vi "mWmotor_Set_Driver_current.vi"(8 "error in (no error)":errorcluster, 10 "Boolean":bool, 11 "VISA resource name":refnum<visa-resource-name>) -> (0 "error out":errorcluster, 3 "VISA resource name out":refnum<visa-resource-name>)   [LabVIEW 2019]
panel:
  in  "milliseconds to wait":u32=100
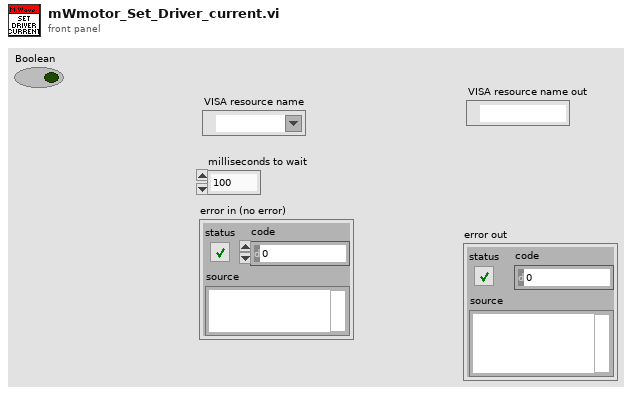
[diagram p1: front panel]
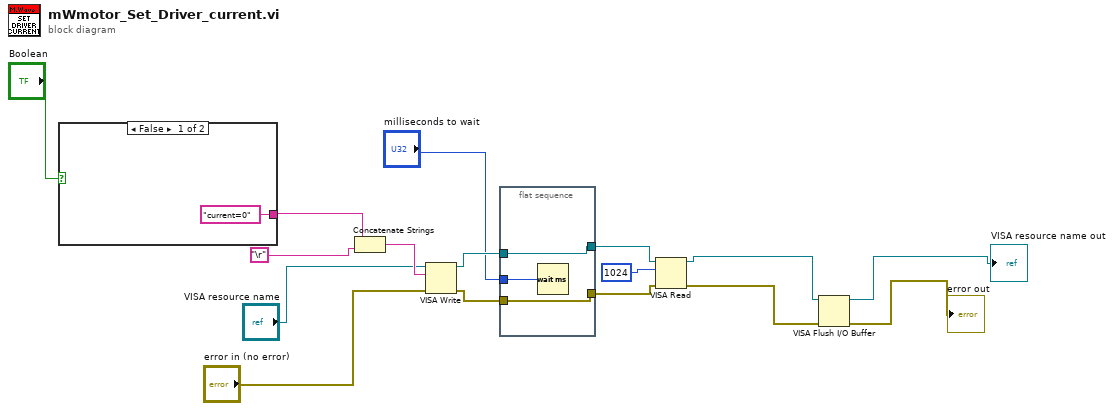
[diagram p0: block diagram]
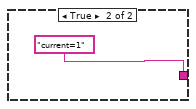
[diagram p2: hidden frame]
diagram:
  n1 = case shown="False" "Boolean" {
    tunnel: ["current=0" ("string") "current=1" ("string")] -> w7
    frame False {
    }
    frame True {
    }
  }
  n2 = Concatenate Strings(w7, "\r") -> (w16:string)
  n3 = VISA Write(VISA resource name="VISA resource name", write buffer=w16, error in (no error)="error in (no error)") -> (VISA resource name out=w12:refnum<visa-resource-name>, error out=w13:errorcluster)  [unwired: 1 out]
  n4 = flat-sequence {
    tunnel: [w21] -> w6
    tunnel: w13 -> [w21]
    tunnel: [w20] -> w11
    tunnel: w12 -> [w20]
    tunnel: "milliseconds to wait" -> [w19]
    frame #0 {
      n5 = Wait (ms)(milliseconds to wait=w19) -> ()  [unwired: 1 out]
    }
  }
  n6 = VISA Read(VISA resource name=w11, byte count=u32 1024, error in (no error)=w6) -> (VISA resource name out=w5:refnum<visa-resource-name>, error out=w3:errorcluster)  [unwired: 2 out]
  n7 = VISA Flush I/O Buffer(VISA resource name=w5, error in (no error)=w3) -> (VISA resource name out=→"VISA resource name out":refnum<visa-resource-name>, error out=→"error out":errorcluster)  [unwired: 1 in]
